vi "Corridor to Diag. Scale.vi"(8 "Command Info In":T2, 9 "Target Height (in)":dbl, 10 "Block Inputs":T1, 11 "Starting Position":T5) -> (0 "Command Info Out":T2)   [LabVIEW 2017]
uses:
  <vilib>/Rock Robotics/WPI/Framework/Command Status Info.ctl
  <vilib>/Rock Robotics/WPI/Framework/Completion Status.ctl
  <vilib>/Rock Robotics/WPI/Framework/Completion Notifier.ctl
  Support Code/Starting Position.ctl
  Support Code/Extended Block Inputs.ctl
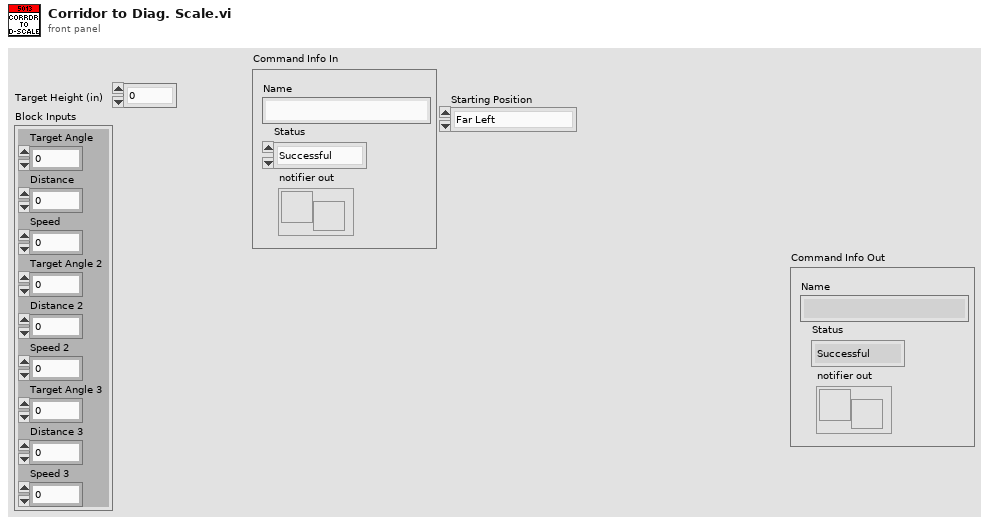
[diagram p1: front panel]
types:
  T1 = typedef "Extended Block Inputs.ctl" = cluster{"Target Angle":dbl, "Distance":dbl, "Speed":dbl, "Target Angle 2":dbl, "Distance 2":dbl, "Speed 2":dbl, "Target Angle 3":dbl, "Distance 3":dbl, "Speed 3":dbl}
  T2 = typedef "Command Status Info.ctl" = cluster{"Name":string, "Status":T3, "notifier out":T4}
  T3 = typedef "Completion Status.ctl" = enum16{"Successful", "Aborted", "Incomplete"}
  T4 = typedef "Completion Notifier.ctl" = refnum<notifier>
  T5 = typedef "Starting Position.ctl" = enum16{"Far Left", "Center", "Far Right"}
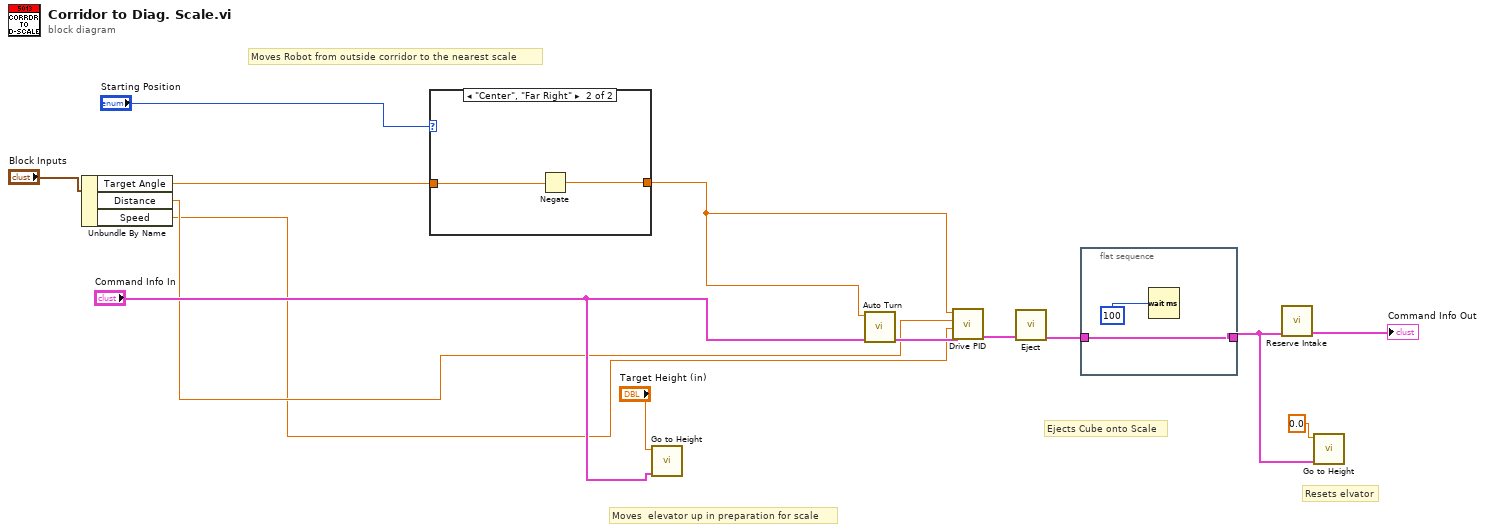
[diagram p0: block diagram]
diagram:
  # "Resets elvator"
  # "Ejects Cube onto Scale"
  # "Moves  elevator up in preparation for scale"
  # "Moves Robot from outside corridor to the nearest scale"
  n1 = Unbundle By Name("Block Inputs") -> ("Target Angle"=w3:dbl, "Distance"=w2:dbl, "Speed"=w1:dbl)
  n2 = case shown="\"Center\", \"Far Right\"" "Starting Position" {
    tunnel: [w15 w17] -> w13
    tunnel: w3 -> [w15 w16]
    frame "Far Left", Default {
    }
    frame "Center", "Far Right" {
      n3 = Negate(x=w16) -> (-x=w17:dbl)
    }
  }
  n4 = call "Go to Height.vi"("Command Info In"="Command Info In", "Target Height (in)"="Target Height (in)") -> ()  [unwired: 9 in, 1 out]
  n5 = call "Auto Turn.vi"("Command Info In"="Command Info In", "Target Angle"=w13) -> ("Command Info Out"=w12:T2)  [unwired: 9 in]
  n6 = call "Drive PID.vi"("Command Info In"=w12, "Speed"=w1, "Distance"=w2, "Target Angle"=w13) -> ("Command Info Out"=w9:T2)  [unwired: 7 in]
  n7 = call "Eject.vi"("Command Info In"=w9) -> ("Command Info Out"=w8:T2)  [unwired: 10 in]
  n8 = flat-sequence {
    tunnel: w8 -> [w18]
    tunnel: [w18] -> w6
    frame #0 {
      n9 = Wait (ms)(milliseconds to wait=u32 100) -> ()  [unwired: 1 out]
    }
  }
  n10 = call "Reserve Intake.vi"("Command Info"=w6) -> ("Command Info"=→"Command Info Out":T2)  [unwired: 10 in]
  n11 = call "Go to Height.vi"("Command Info In"=w6, "Target Height (in)"=0.0) -> ()  [unwired: 9 in, 1 out]
